vi "Debug Test (Send).vi"() -> ()   [LabVIEW 2009]
uses:
  UDP Lib/UDP Network Location.ctl
  Debug Shared/Control Information.ctl
  cRIO/Sensors/Sensor Typedefs/FPGA Main ref.ctl
  cRIO/Sensors/Sensor Typedefs/GPS Data.ctl
  cRIO/Sensors/Sensor Typedefs/SICK Array.ctl
  Remote Control/Motor Command.ctl
  cRIO/Queue Type Def's/Motor State.ctl
  cRIO/Queue Type Def's/Motor Instruction.ctl
  cRIO/Startup VI Support Files/Main State.ctl
  Remote Control/Control Message.ctl
panel:
  in  "Control Info.":T1
  in  "HB 2":bool
  in  "Safety Disabled":bool
  in  "Camera  Init Complete 2":bool
  in  "HB":bool
  in  "Control Message":T2
  in  "RC/!Run":bool=TRUE
  in  "Main State":T4=enum."Remote Control"
  in  "MC VISA resource":refnum<visa-resource-name>="ASRL1::INSTR"
  in  "Motors Init Complete":bool=TRUE
  in  "Motor Queue":refnum<queue>
  in  "RC Command Buffer":T3
  in  "Motors On?":bool=TRUE
  in  "Sensors Init Complete":bool=TRUE
  in  "SICK Buffer":T5
  in  "Compass Buffer":dbl=181.1
  in  "Compass Init Complete":bool
  in  "SICK Init Complete":bool
  in  "GPS Init Complete":bool
  in  "GPS Buffer":T6
  in  "FPGA VI Reference":T7
  in  "Motor Message":string
  in  "VFH Queue":refnum<queue>
  in  "Communication Queue":refnum<queue>
  in  "Camera  Init Complete":bool
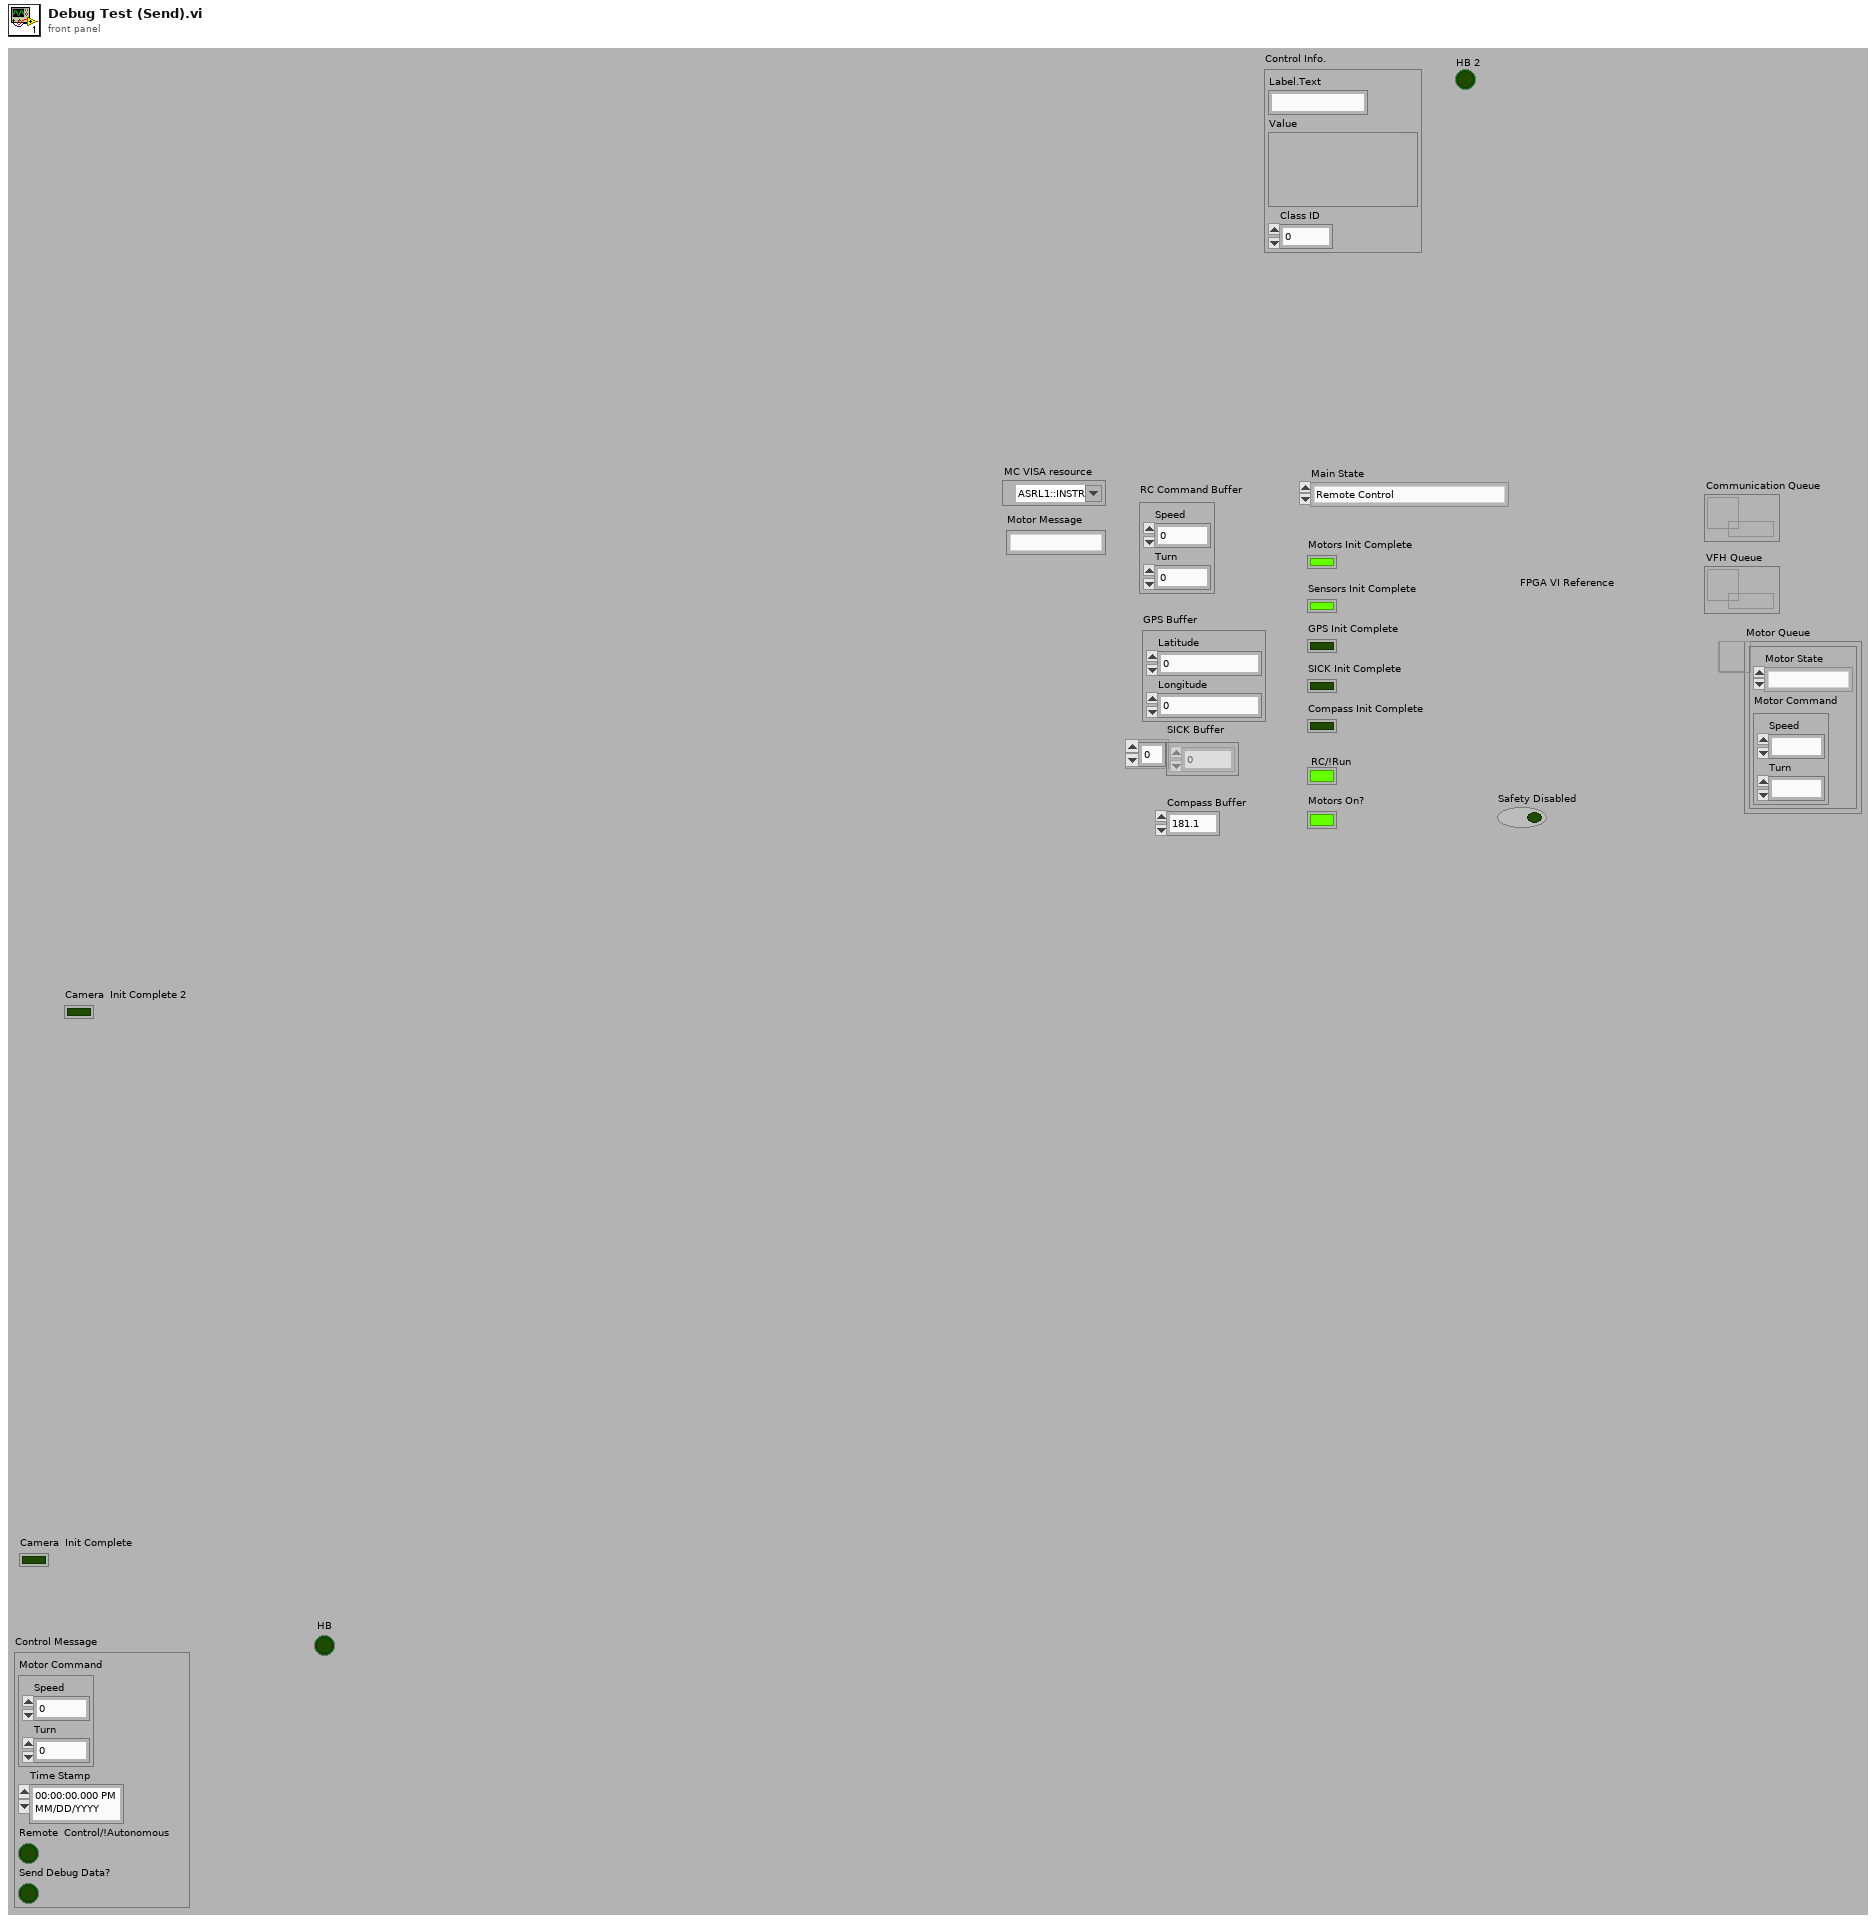
[diagram p1: front panel]
types:
  T1 = typedef "Control Information.ctl" = cluster{"Label.Text":string, "Value":variant, "Class ID":u32}
  T2 = typedef "Control Message.ctl" = cluster{"Motor Command":T3, "Time Stamp":timestamp, "Remote  Control/!Autonomous":bool, "Send Debug Data?":bool}
  T3 = typedef "Motor Command.ctl" = cluster{"Speed":i16, "Turn":i16}
  T4 = typedef "Main State.ctl" = enum16{"Initialize Sensors", "Initialize Motors", "Wait for GO", "Run", "Remote Control", "Stop"}
  T5 = typedef "SICK Array.ctl" = u16[]
  T6 = typedef "GPS Data.ctl" = cluster{"Latitude":dbl, "Longitude":dbl}
  T7 = typedef "FPGA Main ref.ctl" = refnum<k20>
  T8 = typedef "UDP Base.ctl" = cluster{"UDP Session":refnum<k16>, "UDP Socket Params":T9}
  T9 = typedef "UDP Socket Params.ctl" = cluster{"Local Port":u16, "Read Timeout":i32, "Write Timeout":i32}
  T10 = typedef "UDP Network Location.ctl" = cluster{"IP Address":string, "Port":u16}
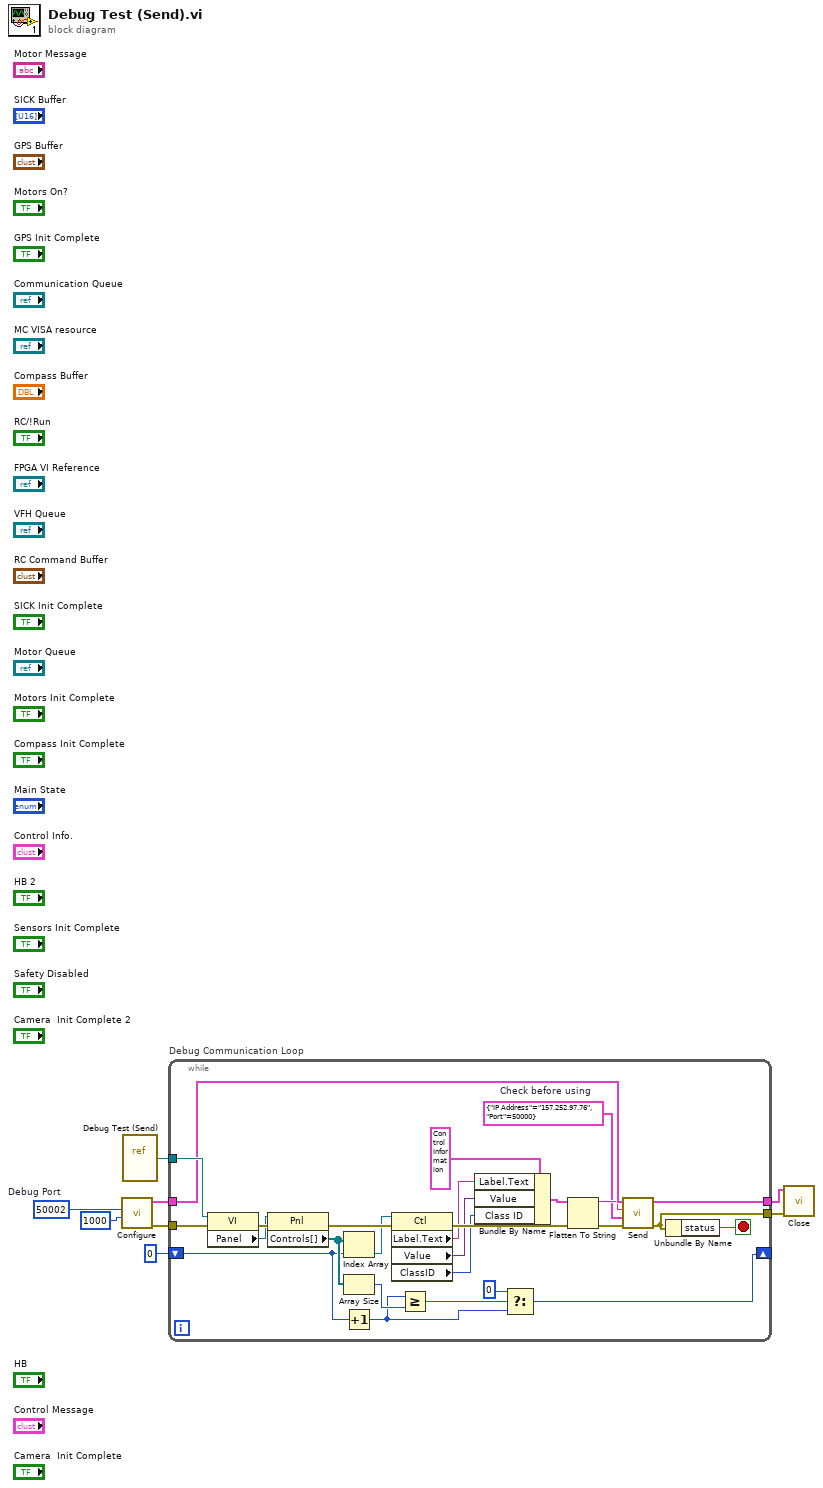
[diagram p0: block diagram]
diagram:
  w7 = u16 50002  # Debug Port
  n1 = call "Configure.vi"("Read Timeout"=1000, "Local Port"=w7) -> ("error out"=w6:errorcluster, "UDP Base out"=w5:T8)  [unwired: 8 in]
  n2 = vi-ref "Debug Test (Send).vi"() -> (w2:refnum<vi>)
  n3 = while "Debug Communication Loop" {
    tunnel: w5 -> [w27]
    tunnel: w6 -> [w28]
    tunnel: [w22] -> w4
    tunnel: [w26] -> w3
    tunnel: w2 -> [w30]
    shift-right: [w10] -> _
    shift-left: 0 ("index") -> [w15]
    stop <- w31 stop-if-true
    w21 = T10 {"IP Address"="157.252.97.76", "Port"=50000}  # Check before using
    n4 = property class="VI"(reference=w30, error in=w28) -> (error out=w34:errorcluster, "Panel"=w33:refnum<vi>)  [unwired: 1 out]
    n5 = property class="Pnl"(reference=w33, error in=w34) -> (error out=w32:errorcluster, "Controls[]"=w16:refnum<vi>[])  [unwired: 1 out]
    n6 = Index Array(array=w16, index=w15) -> (element=w9:refnum<vi>)
    n7 = Array Size(array=w16) -> (size(s)=w14:i32)
    n8 = Increment(x=w15) -> (x+1=w12:i32)
    n9 = property class="Ctl"(reference=w9, error in=w32) -> (error out=w24:errorcluster, "Label.Text"=w19:string, "Value"=w18:variant, "ClassID"=w17:u32)  [unwired: 1 out]
    n10 = Greater Or Equal?(x=w12, y=w14) -> (x >= y?=w13:bool)
    n11 = Bundle By Name(cluster=T1 {"Label.Text"="", "Value"=variant, "Class ID"=0} ("Control Information"), "Label.Text"=w19, "Value"=w18, "Class ID"=w17) -> (w29:T1)
    n12 = Select(t=0, s=w13, f=w12) -> (s? t:f=w10:i32)
    n13 = Flatten To String(anything=w29, error in (no error)=w24) -> (data string=w25:string, error out=w23:errorcluster)  [unwired: 2 in, 1 out]
    n14 = call "Send.vi"("error in (no error)"=w23, "Destination Location"=w21, "Send Data"=w25, "UDP Base in"=w27) -> ("error out"=w22:errorcluster, "UDP Base out"=w26:T8)  [unwired: 5 in, 1 out]
    n15 = Unbundle By Name(w22) -> ("status"=w31:bool)
  }
  n16 = call "Close.vi"("error in (no error)"=w4, "Cluster of class private data"=w3) -> ()  [unwired: 9 in, 1 out]
